vi "Apply Weight.vi"(8 "error in":errorcluster, 9 "Slot Number":i32, 10 "Chuck Number":i32, 11 "GrabberTool in":refnum<class "GrabberTool Class.lvclass">) -> (0 "error out":errorcluster, 3 "GrabberTool out":refnum<class "GrabberTool Class.lvclass">)   [LabVIEW 2011, in "GrabberTool Class.lvclass"]
uses:
  GrabberTool Class.lvclass
  Config Manager Class/Type Definitions/Offset.ctl
  Config Manager Class/Type Definitions/Part Type.ctl
  Config Manager Class/Type Definitions/Named Position.ctl
  WorkTable Class/WorkTable Class.lvclass
  Vec3d Class/Vec3d Class.lvclass
  Config Manager Class/Config Manager Class.lvclass
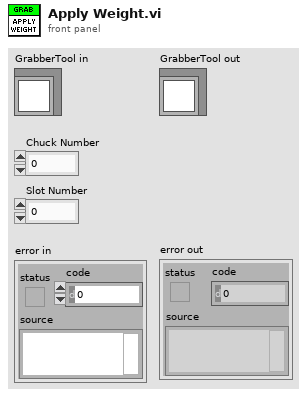
[diagram p1: front panel]
types:
  T1 = enum16{"Empty", "Bare HDI", "Unglued", "Stamped", "PartOnTop", "Weighted", "Unpotted", "Potted"}
  T2 = enum16{"Vertical First", "Lateral First", "Auto"}
  T3 = typedef "Offset.ctl" = enum16{"needle_offset", "tool_holder_offset"}
  T4 = typedef "Part Type.ctl" = enum16{"BBM", "HDI", "BARE HDI", "GLUERESERVOIR", "STAMP_1", "STAMP_2", "STAMP_3", "STAMP_4", "STAMP_5", "WEIGHT_1", "WEIGHT_2", "WEIGHT_3", "WEIGHT_4", "WEIGHT_5", "WEIGHT_6", "WEIGHT_7", "WEIGHT_8", "PICKER_TOOL", "GRABER_TOOL"}
  T5 = typedef "Named Position.ctl" = enum16{"home", "module_chuck_0", "module_chuck_1", "module_chuck_2", "module_chuck_3", "module_chuck_4", "glue_reservoir_chuck", "stamp_tool_chuck", "weight_tool_chuck", "needle_calibration", "tool_rack_pos_0_in", "tool_rack_pos_0_out", "tool_rack_pos_1_in", "tool_rack_pos_1_out", "tool_rack_pos_2_in", "tool_rack_pos_2_out", "front_load_position", "grabber_start_pos", "between_chuck_0_and_1", "between_chuck_2_and_3"}
  T6 = typedef "Worktable_Module Slot.ctl" = cluster{"Slot State":enum16{"Empty", "Bare HDI", "Unglued", "Stamped", "PartOnTop", "Weighted", "Unpotted", "Potted"}, "BBM Type":enum16{"None", "BBM", "GlassSlide"}, "HDI Type":enum16{"None", "HDI", "Polyimide"}, "Vacuum Channel":u8, "Location/Orientation BBM":T7, "Location/Orientation HDI":T7, "S/N":string}
  T7 = typedef "Position_Orientation.ctl" = cluster{"Center":refnum<class "Vec3d Class.lvclass">, "Orientation":refnum<class "Orient3d Class.lvclass">}
  T8 = typedef "Weight Type.ctl" = enum16{"Weight 1", "Weight 2", "Weight 3", "Weight 4", "Weight 5", "Weight 6", "Weight 7", "Weight 8"}
  T9 = typedef "Gluing Parameters.ctl" = cluster{"Safe Grabber Pickup":dbl, "Safe Grabber Lift":dbl, "Glue Resevoir Wait Time":dbl, "Glue BM Wait Time ":dbl, "Placed Weight X-Move":dbl}
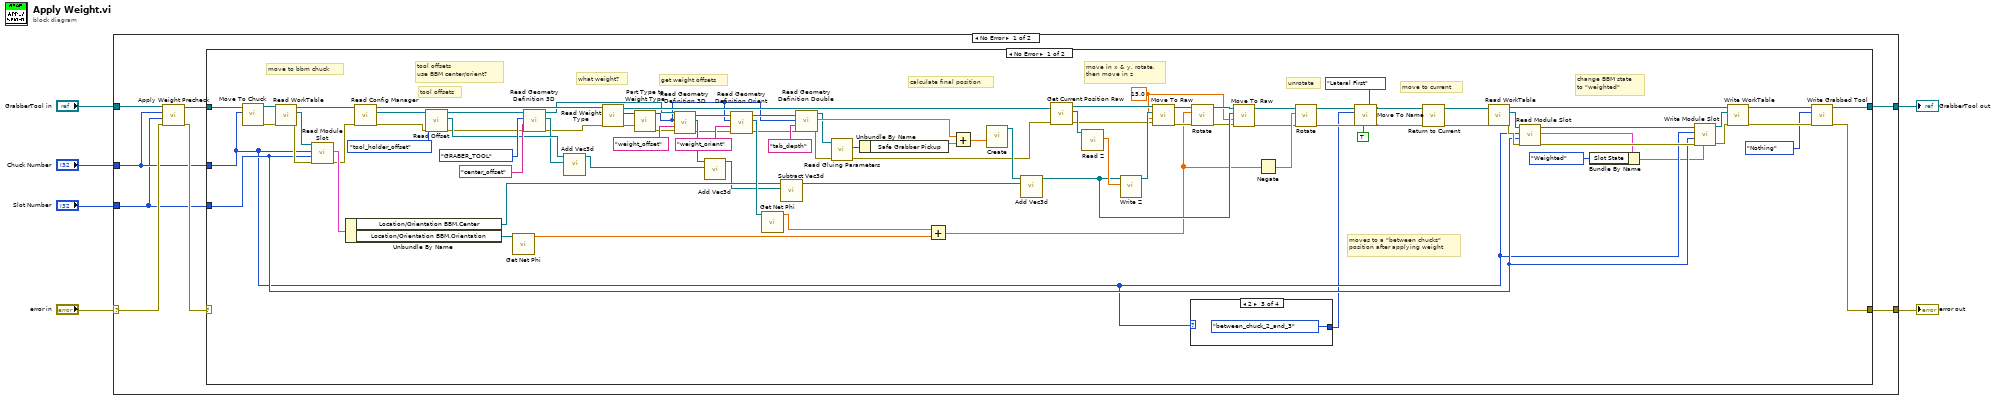
[diagram p0: block diagram]
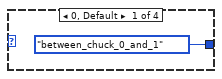
[diagram p2: hidden frame]
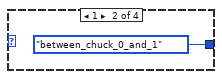
[diagram p3: hidden frame]
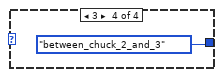
[diagram p4: hidden frame]
diagram:
  n1 = case shown="No Error" "error in" {
    selector: "error in" -> [w10 w112]
    tunnel: [w14 w112] -> w5
    tunnel: [w13 w111] -> w3
    tunnel: "GrabberTool in" -> [w12 w111]
    tunnel: "Chuck Number" -> [w8 _]
    tunnel: "Slot Number" -> [w7 _]
    frame No Error {
      n2 = call "Apply Weight Precheck.vi"("error in (no error)"=w10, "Slot Number"=w7, "Chuck Number"=w8, "GrabberTool Class in"=w12) -> ("error out"=w9:errorcluster, "GrabberTool Class out"=w11:refnum<class "GrabberTool Class.lvclass">)  [unwired: 6 in]
      n3 = case shown="No Error" w9 {
        selector: w9 -> [_ w109]
        tunnel: [w103 w109] -> w14
        tunnel: [w104 w110] -> w13
        tunnel: w11 -> [w85 w110]
        tunnel: w8 -> [w45 _]
        tunnel: w7 -> [w50 _]
        frame No Error {
          w43 = 15.0 ("Speed")
          # "tool offsets"
          # "change BBM state\nto \"weighted\""
          # "move to current"
          # "moves to a \"between chucks\" \nposition after applying weight"
          # "unrotate"
          # "move in x & y, rotate,\nthen move in z"
          # "calculate final position"
          # "get weight offsets"
          # "what weight?"
          # "tool offsets\nuse BBM center/orient?"
          # "move to bbm chuck"
          n4 = call-dynamic "Move To Chuck.vi"("Chuck"=w45, "Gantry in"=w85) -> ("error out"=w86:errorcluster, "Gantry out"=w101:refnum<class "GrabberTool Class.lvclass">)  [unwired: 8 in]
          n5 = call-dynamic "Read WorkTable.vi"("error in"=w86, "Gantry Class in"=w101) -> ("error out"=w87:errorcluster, "WorkTable Class.lvclass"=w100:refnum<class "WorkTable Class.lvclass">, "Gantry Class out"=w99:refnum<class "GrabberTool Class.lvclass">)  [unwired: 7 in]
          n6 = call-dynamic "Read Module Slot.vi"("error in"=w87, "slot"=w50, "chuck"=w45, "WorkTable in"=w100) -> ("error out"=w88:errorcluster, "Module Slot"=w102:T6)  [unwired: 5 in, 1 out]
          n7 = Unbundle By Name(w102) -> ("Location/Orientation BBM.Center"=w20:refnum<class "Vec3d Class.lvclass">, "Location/Orientation BBM.Orientation"=w91:refnum<class "Orient3d Class.lvclass">)
          n8 = call-dynamic "Read Config Manager.vi"("error in"=w88, "Gantry in"=w99) -> ("error out"=w89:errorcluster, "Config Manager"=w98:refnum<class "Config Manager Class.lvclass">, "Gantry out"=w84:refnum<class "GrabberTool Class.lvclass">)  [unwired: 7 in]
          n9 = call "Read Offset.vi"("error in"=w89, "Offset"=Offset."tool_holder_offset", "Config Manager in"=w98) -> ("error out"=w90:errorcluster, "Vec3d out"=w93:refnum<class "Vec3d Class.lvclass">, "Config Manager out"=w95:refnum<class "Config Manager Class.lvclass">)  [unwired: 6 in]
          n10 = call "Get Net Phi.vi"("Orient3d"=w91) -> ("phi(deg)"=w26:dbl)  [unwired: 8 in, 2 out]
          n11 = call "Read Geometry Definition 3D.vi"("error in"=w90, "Feature"="center_offset", "Part Type"=Part_Type."GRABER_TOOL", "Config Manager in"=w95) -> ("error out"=w83:errorcluster, "Feature Coordinates"=w92:refnum<class "Vec3d Class.lvclass">, "Config Manager out"=w35:refnum<class "Config Manager Class.lvclass">)  [unwired: 5 in]
          n12 = call-dynamic "Add Vec3d.vi"(10:"Vec3d Class in"=w92, 11:"Vec3d Class in"=w93) -> ("Vec3d Class out"=w19:refnum<class "Vec3d Class.lvclass">)  [unwired: 8 in, 1 out]
          n13 = call "Read Weight Type.vi"("error in (no error)"=w83, "GrabberTool Class in"=w84) -> ("error out"=w80:errorcluster, "Weight Type"=w82:T8, "GrabberTool Class out"=w74:refnum<class "GrabberTool Class.lvclass">)  [unwired: 7 in]
          n14 = call "Part Type to Weight Type.vi"("error in"=w80, "Weight Type"=w82) -> ("error out"=w22:errorcluster, "Part Type"=w31:T4)  [unwired: 8 in]
          n15 = call "Read Geometry Definition 3D.vi"("error in"=w22, "Feature"="weight_offset", "Part Type"=w31, "Config Manager in"=w35) -> ("error out"=w24:errorcluster, "Feature Coordinates"=w29:refnum<class "Vec3d Class.lvclass">, "Config Manager out"=w33:refnum<class "Config Manager Class.lvclass">)  [unwired: 5 in]
          n16 = call-dynamic "Add Vec3d.vi"(10:"Vec3d Class in"=w19, 11:"Vec3d Class in"=w29) -> ("Vec3d Class out"=w18:refnum<class "Vec3d Class.lvclass">)  [unwired: 8 in, 1 out]
          n17 = call "Read Geometry Definition Orient.vi"("error in"=w24, "Feature"="weight_orient", "Part Type"=w31, "Config Manager in"=w33) -> ("error out"=w23:errorcluster, "Orient3d out"=w28:refnum<class "Orient3d Class.lvclass">, "Config Manager out"=w32:refnum<class "Config Manager Class.lvclass">)  [unwired: 5 in]
          n18 = call "Get Net Phi.vi"("Orient3d"=w28) -> ("phi(deg)"=w27:dbl)  [unwired: 8 in, 2 out]
          n19 = call "Subtract Vec3d.vi"("Vec3d in 2"=w18, "Vec3d in 1"=w20) -> ("Vec3d Class out"=w17:refnum<class "Vec3d Class.lvclass">)  [unwired: 8 in, 1 out]
          n20 = call "Read Geometry Definition Double.vi"("error in"=w23, "Feature"="tab_depth", "Part Type"=w31, "Config Manager in"=w32) -> ("error out"=w36:errorcluster, "Geometry Definition"=w77:dbl, "Config Manager out"=w37:refnum<class "Config Manager Class.lvclass">)  [unwired: 5 in]
          n21 = call "Read Gluing Parameters.vi"("error in (no error)"=w36, "Config Manager Class in"=w37) -> ("error out"=w64:errorcluster, "Gluing Parameters"=w79:T9)  [unwired: 7 in, 1 out]
          n22 = Unbundle By Name(w79) -> ("Safe Grabber Pickup"=w78:dbl)
          n23 = Add(x=w27, y=w26) -> (x+y=w25:dbl)
          n24 = Add(x=w77, y=w78) -> (x+y=w76:dbl)
          n25 = call "Create.vi"("Z"=w76) -> ("Vec3d Class out"=w75:refnum<class "Vec3d Class.lvclass">)  [unwired: 9 in, 1 out]
          n26 = call-dynamic "Add Vec3d.vi"(10:"Vec3d Class in"=w17, 11:"Vec3d Class in"=w75) -> ("Vec3d Class out"=w67:refnum<class "Vec3d Class.lvclass">)  [unwired: 8 in, 1 out]
          n27 = call-dynamic "Get Current Position Raw.vi"("error in"=w64, "Gantry in"=w74) -> ("error out"=w63:errorcluster, "Vec3d Class out"=w73:refnum<class "Vec3d Class.lvclass">, "Gantry out"=w71:refnum<class "GrabberTool Class.lvclass">)  [unwired: 7 in]
          n28 = call-dynamic "Read Z.vi"("Vec3d Class in"=w73) -> ("Z"=w72:dbl)  [unwired: 8 in, 2 out]
          n29 = call-dynamic "Write Z.vi"("Z"=w72, "Vec3d Class in"=w67) -> ("Vec3d Class out"=w70:refnum<class "Vec3d Class.lvclass">)  [unwired: 8 in, 1 out]
          n30 = call-dynamic "Move To Raw.vi"("error in"=w63, "Speed"=w43, "Destination"=w70, "Gantry in"=w71) -> ("error out"=w62:errorcluster, "Gantry out"=w69:refnum<class "GrabberTool Class.lvclass">)  [unwired: 6 in]
          n31 = case shown="2" w45 {
            tunnel: [Named_Position."between_chuck_0_and_1" ("Destination") Named_Position."between_chuck_0_and_1" ("Destination") Named_Position."between_chuck_2_and_3" ("Destination") Named_Position."between_chuck_2_and_3" ("Destination")] -> w44
            frame 0, Default {
            }
            frame 1 {
            }
            frame 2 {
            }
            frame 3 {
            }
          }
          n32 = call-dynamic "Rotate.vi"("error in"=w62, "distance(deg)"=w25, "Gantry in"=w69) -> ("error out"=w61:errorcluster, "Gantry out"=w68:refnum<class "GrabberTool Class.lvclass">)  [unwired: 7 in]
          n33 = call-dynamic "Move To Raw.vi"("error in"=w61, "Speed"=w43, "Destination"=w67, "Gantry in"=w68) -> ("error out"=w60:errorcluster, "Gantry out"=w65:refnum<class "GrabberTool Class.lvclass">)  [unwired: 6 in]
          n34 = Negate(x=w25) -> (-x=w66:dbl)
          n35 = call-dynamic "Rotate.vi"("error in"=w60, "distance(deg)"=w66, "Gantry in"=w65) -> ("error out"=w46:errorcluster, "Gantry out"=w47:refnum<class "GrabberTool Class.lvclass">)  [unwired: 7 in]
          n36 = call-dynamic "Move To Name.vi"("Motion Order"=T2."Lateral First", "Direct"=TRUE, "error in"=w46, "Destination"=w44, "Gantry in"=w47) -> ("error out"=w49:errorcluster, "Gantry out"=w48:refnum<class "GrabberTool Class.lvclass">)  [unwired: 5 in]
          n37 = call-dynamic "Return to Current.vi"("error in"=w49, "Gantry in"=w48) -> ("error out"=w51:errorcluster, "Gantry out"=w52:refnum<class "GrabberTool Class.lvclass">)  [unwired: 8 in]
          n38 = call-dynamic "Read WorkTable.vi"("error in"=w51, "Gantry Class in"=w52) -> ("error out"=w54:errorcluster, "WorkTable Class.lvclass"=w59:refnum<class "WorkTable Class.lvclass">, "Gantry Class out"=w58:refnum<class "GrabberTool Class.lvclass">)  [unwired: 7 in]
          n39 = call-dynamic "Read Module Slot.vi"("error in"=w54, "slot"=w50, "chuck"=w45, "WorkTable in"=w59) -> ("error out"=w55:errorcluster, "Module Slot"=w42:T6, "WorkTable out"=w53:refnum<class "WorkTable Class.lvclass">)  [unwired: 5 in]
          n40 = Bundle By Name(cluster=w42, "Slot State"=T1."Weighted") -> (w41:T6)
          n41 = call-dynamic "Write Module Slot.vi"("Module Slot"=w41, "error in"=w55, "slot"=w50, "chuck"=w45, "WorkTable in"=w53) -> ("error out"=w56:errorcluster, "WorkTable out"=w57:refnum<class "WorkTable Class.lvclass">)  [unwired: 5 in]
          n42 = call-dynamic "Write WorkTable.vi"("error in (no error)"=w56, "WorkTable Class.lvclass"=w57, "Gantry Class in"=w58) -> ("error out"=w39:errorcluster, "Gantry Class out"=w40:refnum<class "GrabberTool Class.lvclass">)  [unwired: 7 in]
          n43 = call "Write Grabbed Tool.vi"("error in (no error)"=w39, "Grabbed Tool"=enum16{"Weight Tool", "Stamp Tool", "Nothing"}."Nothing", "GrabberTool Class in"=w40) -> ("error out"=w103:errorcluster, "GrabberTool Class out"=w104:refnum<class "GrabberTool Class.lvclass">)  [unwired: 7 in]
        }
        frame Error {
        }
      }
    }
    frame Error {
    }
  }
  "error out" <- w5
  "GrabberTool out" <- w3
